vi "Update Annotations.vi"(6 "Sample Period":dbl, 8 "Commands":cluster{"Time (s)":dbl, T1, "Enabled":bool}[](array[cluster]), 9 "Trajectory Data":T4(array[cluster]), 10 "Robot Pt Index":i32) -> (1 "Redraw":bool, 2 "Velocity Trace":dbl[](array[numeric]), 3 "Annotation Data":T3(array[cluster]))   [LabVIEW 2019]
uses:
  Command Stuff/Single Cmd Info.ctl
  <vilib>/picture/picture.llb/imagedata.ctl
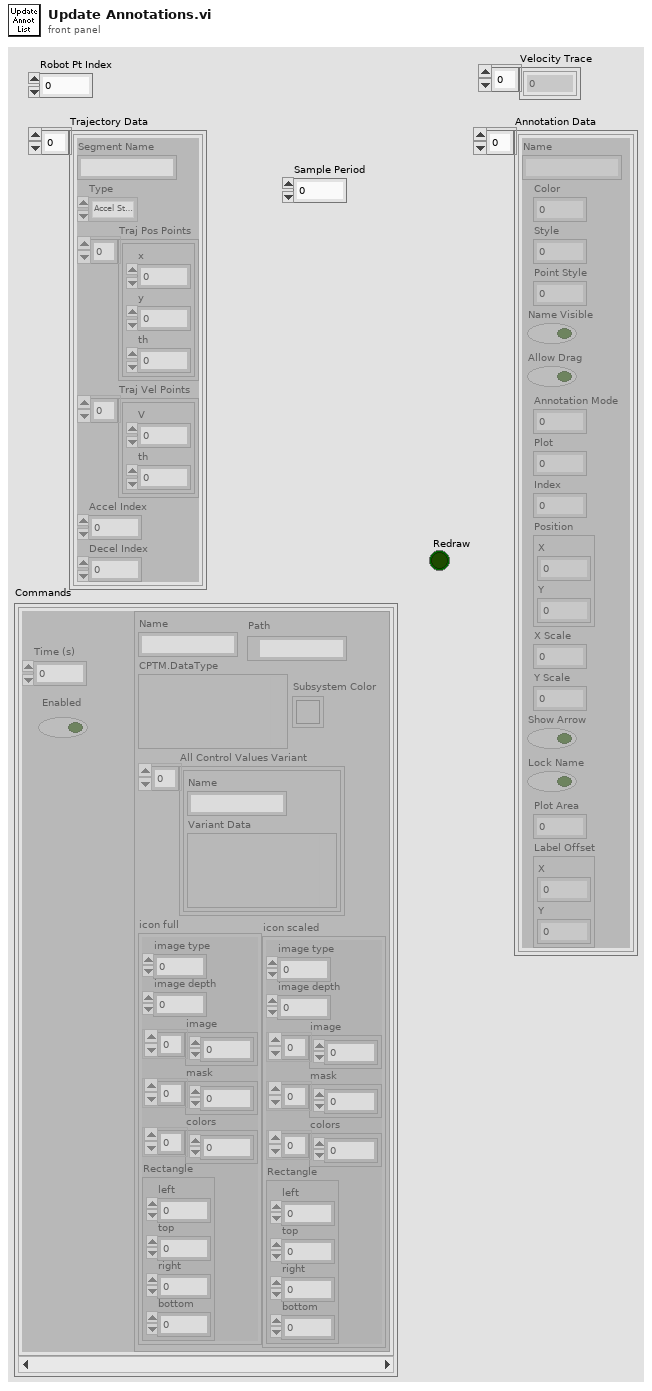
[diagram p1: front panel]
types:
  T1 = typedef "Single Cmd Info.ctl" = cluster{"Name":string, "CPTM.DataType":variant, "All Control Values Variant":cluster{"Name":string, "Variant Data":variant}[], "icon full":T2, "icon scaled":T2, "Path":path, "Subsystem Color":u32}
  T2 = typedef "imagedata.ctl" = cluster{"image type":i32, "image depth":i32, "image":u8[], "mask":u8[], "colors":u32[], "Rectangle":cluster{"left":i16, "top":i16, "right":i16, "bottom":i16}}
  T3 = cluster{"Name":string, "Color":u32, "Style":i32, "Point Style":i32, "Name Visible":bool, "Allow Drag":bool, "Annotation Mode":i32, "Plot":i32, "Index":i32, "Position":cluster{"X":dbl, "Y":dbl}, "X Scale":i32, "Y Scale":u32, "Show Arrow":bool, "Lock Name":bool, "Plot Area":i32, "Label Offset":cluster{"X":dbl, "Y":dbl}}[]
  T4 = cluster{"Segment Name":string, "Type":enum16{"Accel Straight", "Const Straight", "Blend", "Circle"}, "Traj Pos Points":cluster{"x":dbl, "y":dbl, "th":dbl}[], "Traj Vel Points":cluster{"V":dbl, "th":dbl}[], "Accel Index":i32, "Decel Index":i32}[]
  T5 = cluster{"Name":string, "Color":u32, "Style":i32, "Point Style":i32, "Name Visible":bool, "Allow Drag":bool, "Annotation Mode":i32, "Plot":i32, "Index":i32, "Position":cluster{"X":dbl, "Y":dbl}, "X Scale":i32, "Y Scale":u32, "Show Arrow":bool, "Lock Name":bool, "Plot Area":i32, "Label Offset":cluster{"X":dbl, "Y":i32}}
  T6 = enum16{"Accel Straight", "Const Straight", "Blend", "Circle"}
  T7 = cluster{"Name":string, "Color":u32, "Style":i32, "Point Style":i32, "Name Visible":bool, "Allow Drag":bool, "Annotation Mode":i32, "Plot":i32, "Index":i32, "Position":cluster{"X":dbl, "Y":dbl}, "X Scale":i32, "Y Scale":u32, "Show Arrow":bool, "Lock Name":bool, "Plot Area":i32, "Label Offset":cluster{"X":dbl, "Y":i32}}[]
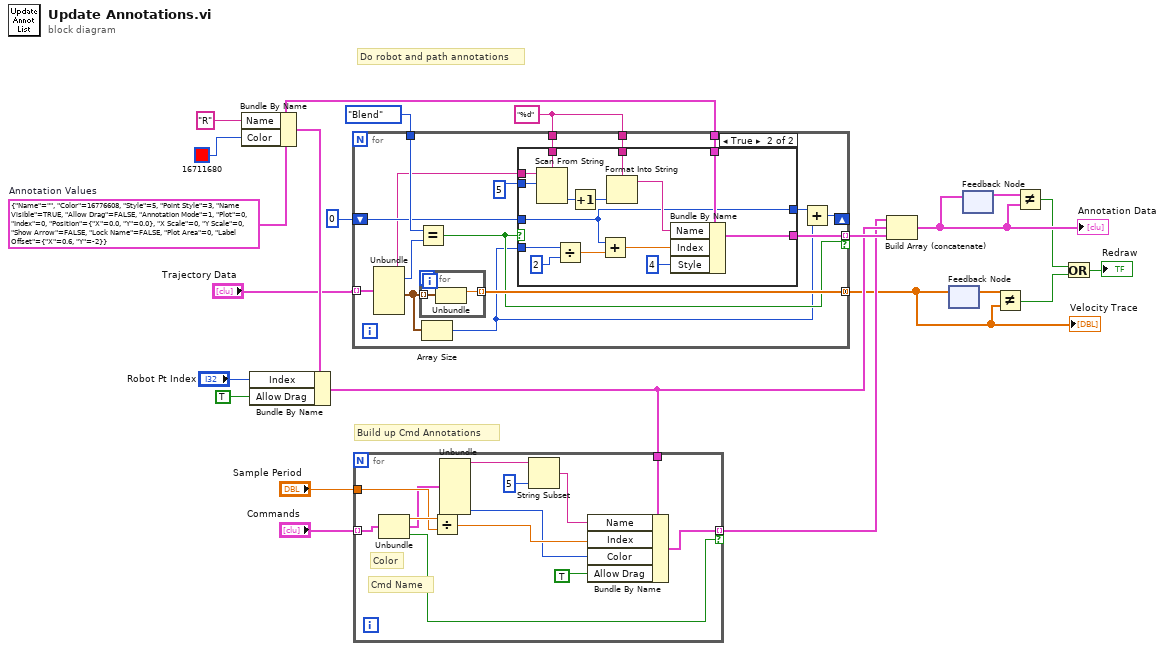
[diagram p0: block diagram]
diagram:
  w13 = T5 {"Name"="", "Color"=16776608, "Style"=5, "Point Style"=3, "Name Visible"=TRUE, "Allow Drag"=FALSE, "Annotation Mode"=1, "Plot"=0, "Index"=0, "Position"={"X"=0.0, "Y"=0.0}, "X Scale"=0, "Y Scale"=0, "Show Arrow"=FALSE, "Lock Name"=FALSE, "Plot Area"=0, "Label Offset"={"X"=0.6, "Y"=-2}}  # Annotation Values
  w16 = "%d" ("Name")
  # "Do robot and path annotations"
  # "Build up Cmd Annotations"
  n1 = Bundle By Name(cluster=w13, "Name"="R", "Color"=u32 16711680) -> (w22:T5)
  n2 = Bundle By Name(cluster=w22, "Index"="Robot Pt Index", "Allow Drag"=TRUE ("Name Visible")) -> (w10:T5)
  n3 = for {
    tunnel: "Trajectory Data" -> [w38] mode=indexing
    tunnel: [w37] -> w4 mode=concatenating
    tunnel: T6."Blend" ("Type") -> [w36]
    shift-right: [w25] -> _
    shift-left: 0 -> [w33]
    tunnel: [w28] -> w18 mode=indexing if=w27
    tunnel: w13 -> [w32]
    tunnel: w16 -> [w30]
    tunnel: w16 -> [w29]
    n4 = Unbundle(w38) -> ("Segment Name"=w31:string, "Type"=w35:T6, "Traj Vel Points"=w34:cluster{"V":dbl, "th":dbl}[])  [unwired: 3 out]
    n5 = Equal?(x=w36, y=w35) -> (x = y?=w27:bool)
    n6 = for {
      tunnel: w34 -> [w56] mode=indexing
      tunnel: [w55] -> w37 mode=indexing
      n7 = Unbundle(w56) -> ("V"=w55:dbl)  [unwired: 1 out]
    }
    n8 = Array Size(array=w34) -> (size(s)=w24:i32)
    n9 = case shown="True" w27 {
      tunnel: w33 -> [w39 w48]
      tunnel: [w39 w48] -> w26
      tunnel: w32 -> [_ w54]
      tunnel: w31 -> [_ w53]
      tunnel: w30 -> [_ w52]
      tunnel: w29 -> [_ w51]
      tunnel: [_ w49] -> w28
      tunnel: w24 -> [_ w45]
      tunnel: 5 -> [_ w44]
      frame False {
      }
      frame True {
        n10 = Scan From String(format string=w52, input string=w53, initial scan location=w44) -> (output 1=w42:i32)  [unwired: 2 in, 3 out]
        n11 = Divide(x=w45, y=2) -> (x/y=w46:dbl)
        n12 = Increment(x=w42) -> (x+1=w41:i32)
        n13 = Add(x=w48, y=w46) -> (x+y=w43:dbl)
        n14 = Format Into String(format string=w51, w41) -> (resulting string=w50:string)  [unwired: 2 in, 1 out]
        n15 = Bundle By Name(cluster=w54, "Name"=w50, "Index"=w43, "Style"=4) -> (w49:T5)
      }
    }
    n16 = Add(x=w26, y=w24) -> (x+y=w25:i32)
  }
  "Velocity Trace" <- w4
  n17 = for {
    tunnel: "Commands" -> [w69] mode=indexing
    tunnel: w10 -> [w68]
    tunnel: [w67] -> w9 mode=indexing if=w61
    tunnel: "Sample Period" -> [w65]
    # "Cmd Name"
    # "Color"
    n18 = Unbundle(w69) -> ("Time (s)"=w66:dbl, w62:T1, "Enabled"=w61:bool)
    n19 = Divide(x=w66, y=w65) -> (x/y=w64:dbl)
    n20 = Unbundle(w62) -> ("Name"=w60:string, "Subsystem Color"=w57:u32)  [unwired: 5 out]
    n21 = String Subset(string=w60, length (rest)=5 ("length (rest)")) -> (substring=w58:string)  [unwired: 1 in]
    n22 = Bundle By Name(cluster=w68, "Name"=w58, "Index"=w64, "Color"=w57, "Allow Drag"=TRUE ("Name Visible")) -> (w67:T5)
  }
  n23 = Build Array (concatenate)(w9, w10, w18) -> (w6:T7)
  "Annotation Data" <- w6
  n24 = feedback #1() -> (w5:dbl[])  [unwired: 1 in]
  n25 = feedback-in #1(w4) -> ()
  n26 = feedback-in #2(w6) -> ()
  n27 = feedback #2() -> (w7:T7)  [unwired: 1 in]
  n28 = Not Equal?(x=w5, y=w4) -> (x != y?=w2:bool)
  n29 = Not Equal?(x=w7, y=w6) -> (x != y?=w3:bool)
  n30 = Or(x=w3, y=w2) -> (x .or. y?=→"Redraw":bool)
